vi "Init_Instr.vi"(8 "error in (no error)":errorcluster caption="entrée d'erreur (pas d'erreur)", 11 "Class Instrument Multimeter en entrée":refnum<class "Class Instrument Balance.lvclass">) -> (0 "error out":errorcluster caption="sortie d'erreur", 3 "Class Instrument Multimeter en sortie":refnum<class "Class Instrument Balance.lvclass">)   [LabVIEW 2020, in "Library Instrument & Equipement.lvlib" / "Library Instruments.lvlib" / "Class Instrument Balance.lvclass"]
uses:
  Class Instrument Balance.lvclass
  Class Instrument Balance.lvclass/Class Instrument Balance.ctl
  Instrument (Default)/Class Instrument (Default).lvclass
  Balance/Balance (Default)/Class Balance (Default).lvclass
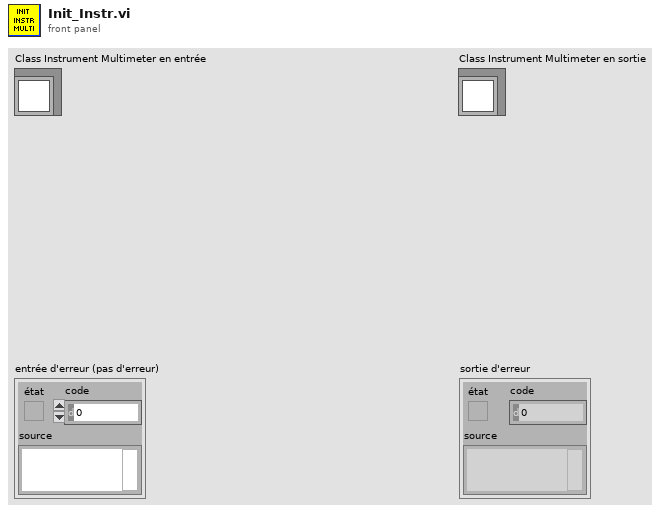
[diagram p1: front panel]
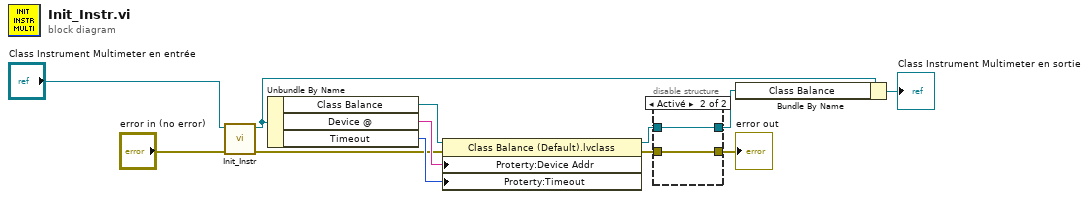
[diagram p0: block diagram]
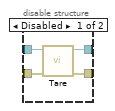
[diagram p2: hidden frame]
diagram:
  n1 = call-parent "Init_Instr.vi"("error in (no error)"="error in (no error)", "Class Instrument (Default) en entrée"="Class Instrument Multimeter en entrée") -> ("error out"=w7:errorcluster, "Class Instrument (Default) en sortie"=w5:refnum<class "Class Instrument Balance.lvclass">)  [unwired: 8 in]
  n2 = Unbundle By Name(w5) -> ("Class Balance"=w10:refnum<class "Class Balance (Default).lvclass">, "Device @"=w9:string, "Timeout"=w8:u32)
  n3 = property class="Class Balance (Default).lvclass"(reference=w10, error in=w7, "Proterty:Device Addr"=w9, "Proterty:Timeout"=w8) -> (reference out=w1:refnum<class "Class Balance (Default).lvclass">, error out=w4:errorcluster)
  n4 = disable-structure shown="Activé" {
    disable-tunnel: w4 -> [w16 w17]
    disable-tunnel: [w15 w17] -> w3
    disable-tunnel: [w14 w18] -> w2
    disable-tunnel: w1 -> [w13 w18]
    frame Disabled {
      n5 = call-dynamic "Tare.vi"("error in (no error)"=w16, "Class Balance (Default) en entrée"=w13) -> ("error out"=w15:errorcluster, "Class Balance (Default) en sortie"=w14:refnum<class "Class Balance (Default).lvclass">)  [unwired: 8 in]
    }
    frame Enabled {
    }
  }
  "error out" <- w3
  n6 = Bundle By Name(cluster=w5, "Class Balance"=w2) -> (→"Class Instrument Multimeter en sortie":refnum<class "Class Instrument Balance.lvclass">)
